vi "Frame_Trigger_Synchronization.vi"() -> ()   [LabVIEW 2016]
panel:
  out "Number of Flashes":dbl
  in  "Frame Number to Sync":dbl=100.0
  in  "stop 2":bool
  out "Trigger Frames":u32
  in  "Loop Time (ms)":u32=10
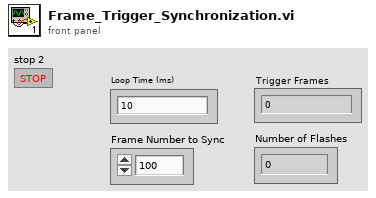
[diagram p1: front panel]
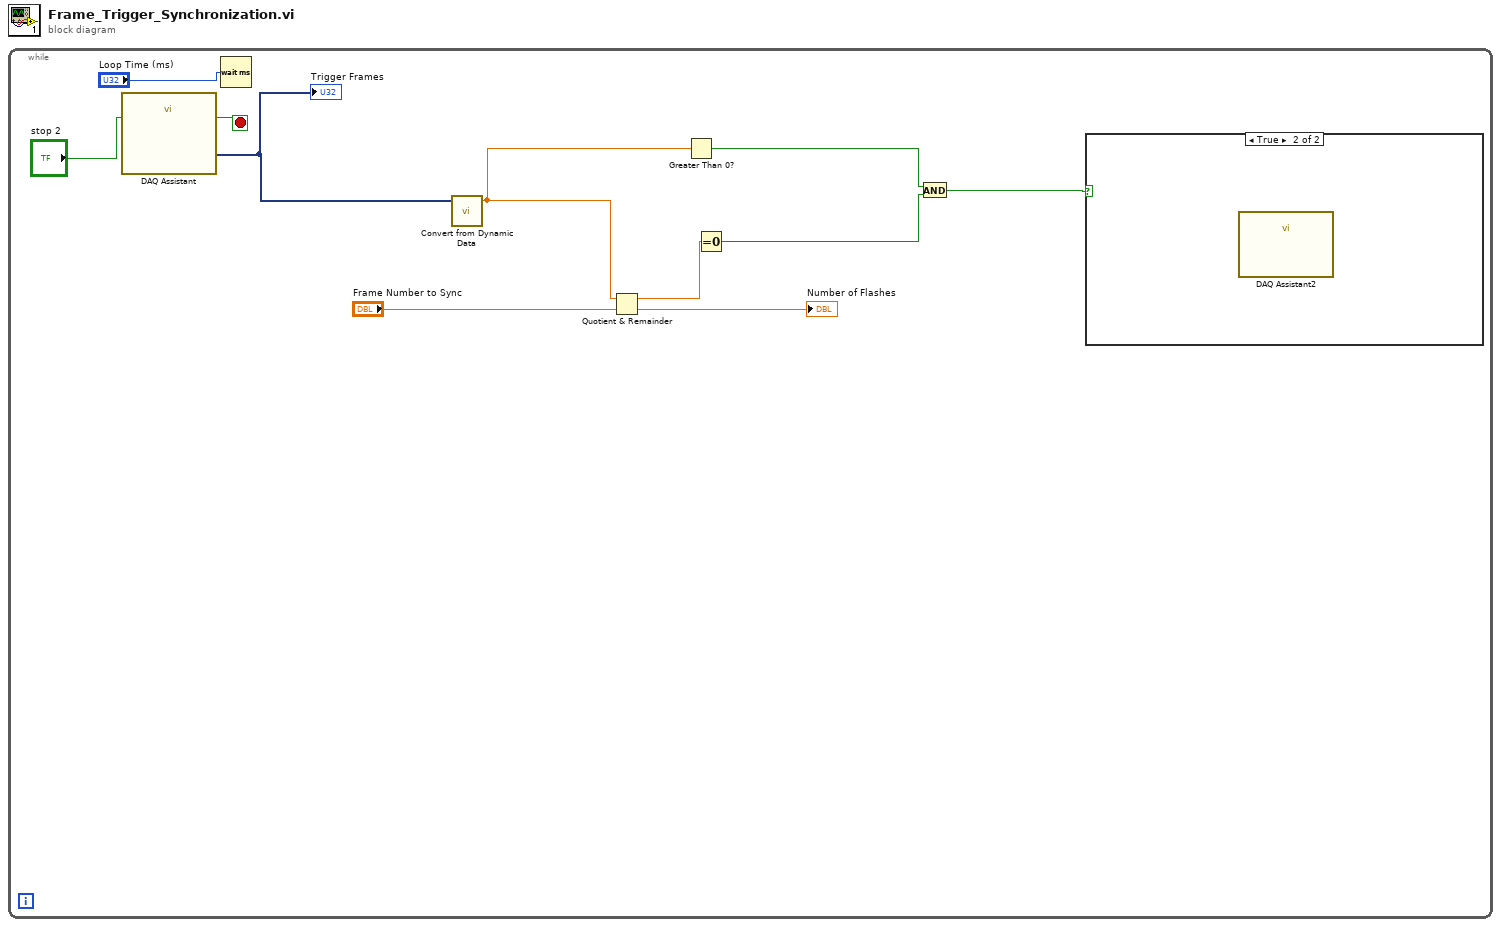
[diagram p0: block diagram]
diagram:
  n1 = while {
    stop <- w11 stop-if-true
    n2 = call "DAQ Assistant"("stop (F)"="stop 2") -> ("data"=w7:dynamicdata, "stopped"=w11:bool)  [unwired: 15 in, 2 out]
    "Trigger Frames" <- w7
    n3 = Wait (ms)(milliseconds to wait="Loop Time (ms)") -> ()  [unwired: 1 out]
    n4 = call "Convert from Dynamic Data"("Dynamic Data Type"=w7) -> ("Scalar"=w1:dbl)  [unwired: 3 in]
    n5 = Quotient & Remainder(x=w1, y="Frame Number to Sync") -> (x-y*floor(x/y)=w3:dbl, floor(x/y)=→"Number of Flashes":dbl)
    n6 = Greater Than 0?(x=w1) -> (x > 0?=w4:bool)
    n7 = Equal To 0?(x=w3) -> (x = 0?=w5:bool)
    n8 = And(x=w4, y=w5) -> (x .and. y?=w6:bool)
    n9 = case shown="True" w6 {
      frame False {
      }
      frame True {
        n10 = call "DAQ Assistant2"() -> ()  [unwired: 18 in, 2 out]
      }
    }
  }
